vi "Replase ALR_ON_OFF consumer.vi"(9 "Data":bool[](array[boolean]), 10 "Index":i32[](array[numeric]), 11 "ALR_ON_OFF":refnum<data-value>) -> (3 "ALR_ON_OFF out":refnum<data-value>)   [LabVIEW 2019]
panel:
  out "error out":errorcluster
  in  "error in (no error)":errorcluster
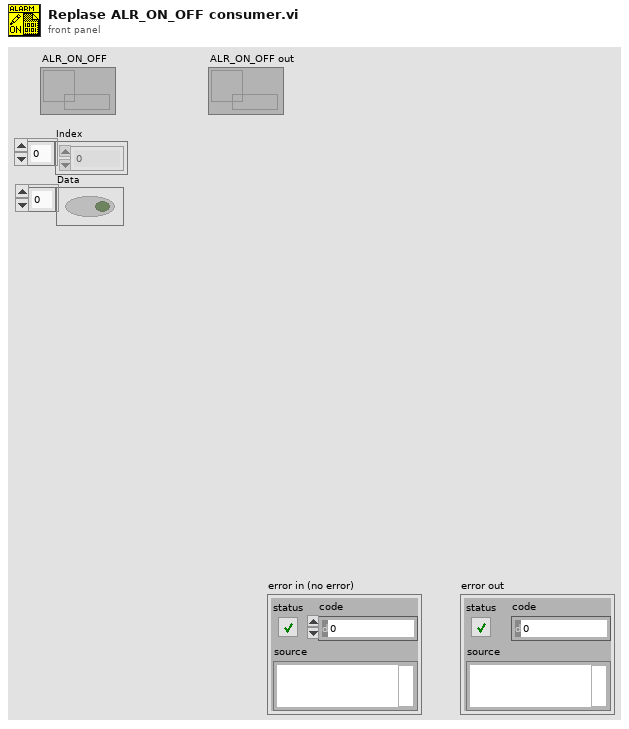
[diagram p1: front panel]
types:
  T1 = cluster{"ALR_ON":bool[], "ALR_OFF":bool[], "ALR_reset":bool[], "ALR_check":bool[], "ALR_block":bool[], "ALR_Ack":bool[]}
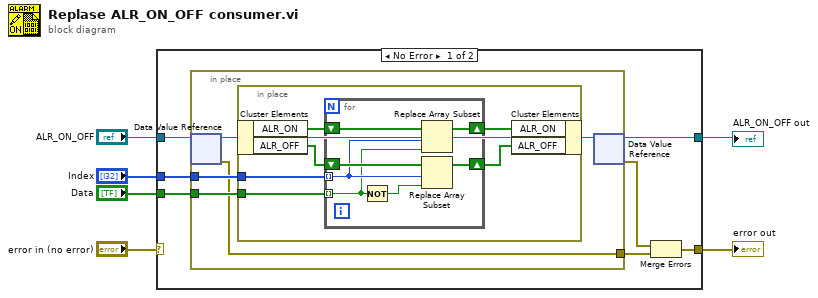
[diagram p0: block diagram]
diagram:
  n1 = case shown="No Error" "error in (no error)" {
    selector: "error in (no error)" -> [_ w32]
    tunnel: "Index" -> [w12 _]
    tunnel: [w7 w32] -> w5
    tunnel: "ALR_ON_OFF" -> [w11 w31]
    tunnel: [w11 w31] -> w2
    tunnel: "Data" -> [w10 _]
    frame No Error {
      n2 = in-place {
        in-place-border: w12 -> [w16]
        in-place-border: w10 -> [w15]
        in-place-border: [w13] -> w8
        n3 = in-place-dvr #1(w11) -> (w17:T1, w13:errorcluster)
        n4 = in-place {
          in-place-border: w16 -> [w22]
          in-place-border: w15 -> [w20]
          n5 = in-place-cluster #2(w17) -> ("ALR_ON"=w23:bool[], "ALR_OFF"=w21:bool[])
          n6 = for {
            tunnel: w22 -> [w28] mode=indexing
            tunnel: w20 -> [w27] mode=indexing
            shift-right: [w26] -> w19
            shift-left: w23 -> [w30]
            shift-right: [w25] -> w18
            shift-left: w21 -> [w29]
            n7 = Not(x=w27) -> (.not. x?=w24:bool)
            n8 = Replace Array Subset(array=w30, new element=w27, index=w28) -> (w26:bool[])
            n9 = Replace Array Subset(array=w29, new element=w24, index=w28) -> (w25:bool[])
          }
          n10 = in-place-cluster #2("ALR_ON"=w19, "ALR_OFF"=w18) -> (w14:T1)
        }
        n11 = in-place-dvr #1(w14) -> (w9:errorcluster)  [unwired: 1 out]
      }
      n12 = Merge Errors(w9, w8) -> (w7:errorcluster)
    }
    frame Error {
    }
  }
  "error out" <- w5
  "ALR_ON_OFF out" <- w2
